vi "LinSpace.vi"   [LabVIEW 2020]
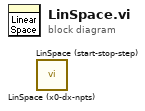
[diagram p0: block diagram]
diagram:
  n1 = call "LinSpace (x0-dx-npts).vi"() -> ()  [unwired: 4 in, 2 out]
  n2 = call "LinSpace (start-stop-step).vi"() -> ()  [unwired: 4 in, 2 out]
